vi "main.vi"() -> ()   [LabVIEW 2019]
uses:
  <vilib>/Utility/file.llb/Write Delimited Spreadsheet (string).vi
  <vilib>/Utility/file.llb/Read Delimited Spreadsheet (DBL).vi
panel:
  in  "设备名":tag="Dev11"
  out "行":i32
  out "列":i32
  in  "?":bool
  out "Log":string
  out "Load6":bool
  out "Load5":bool
  out "Load4":bool
  out "Load3":bool
  out "Load2":bool
  out "Load1":bool
  out "Load0":bool
  out "data":bool[](array[boolean]) caption="数据"
  # "测试报告状态："
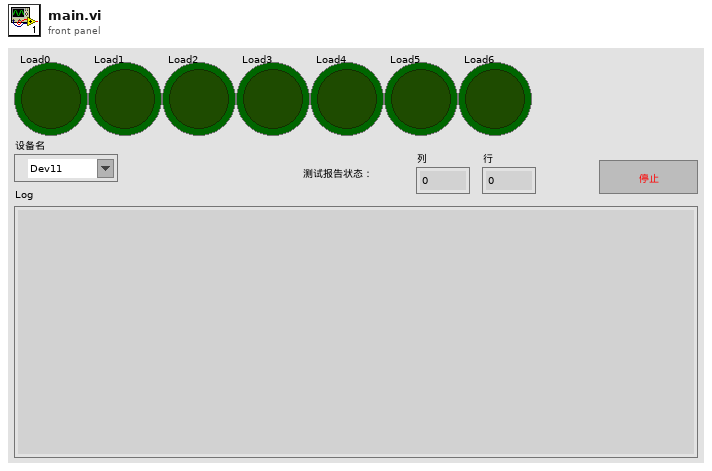
[diagram p1: front panel]
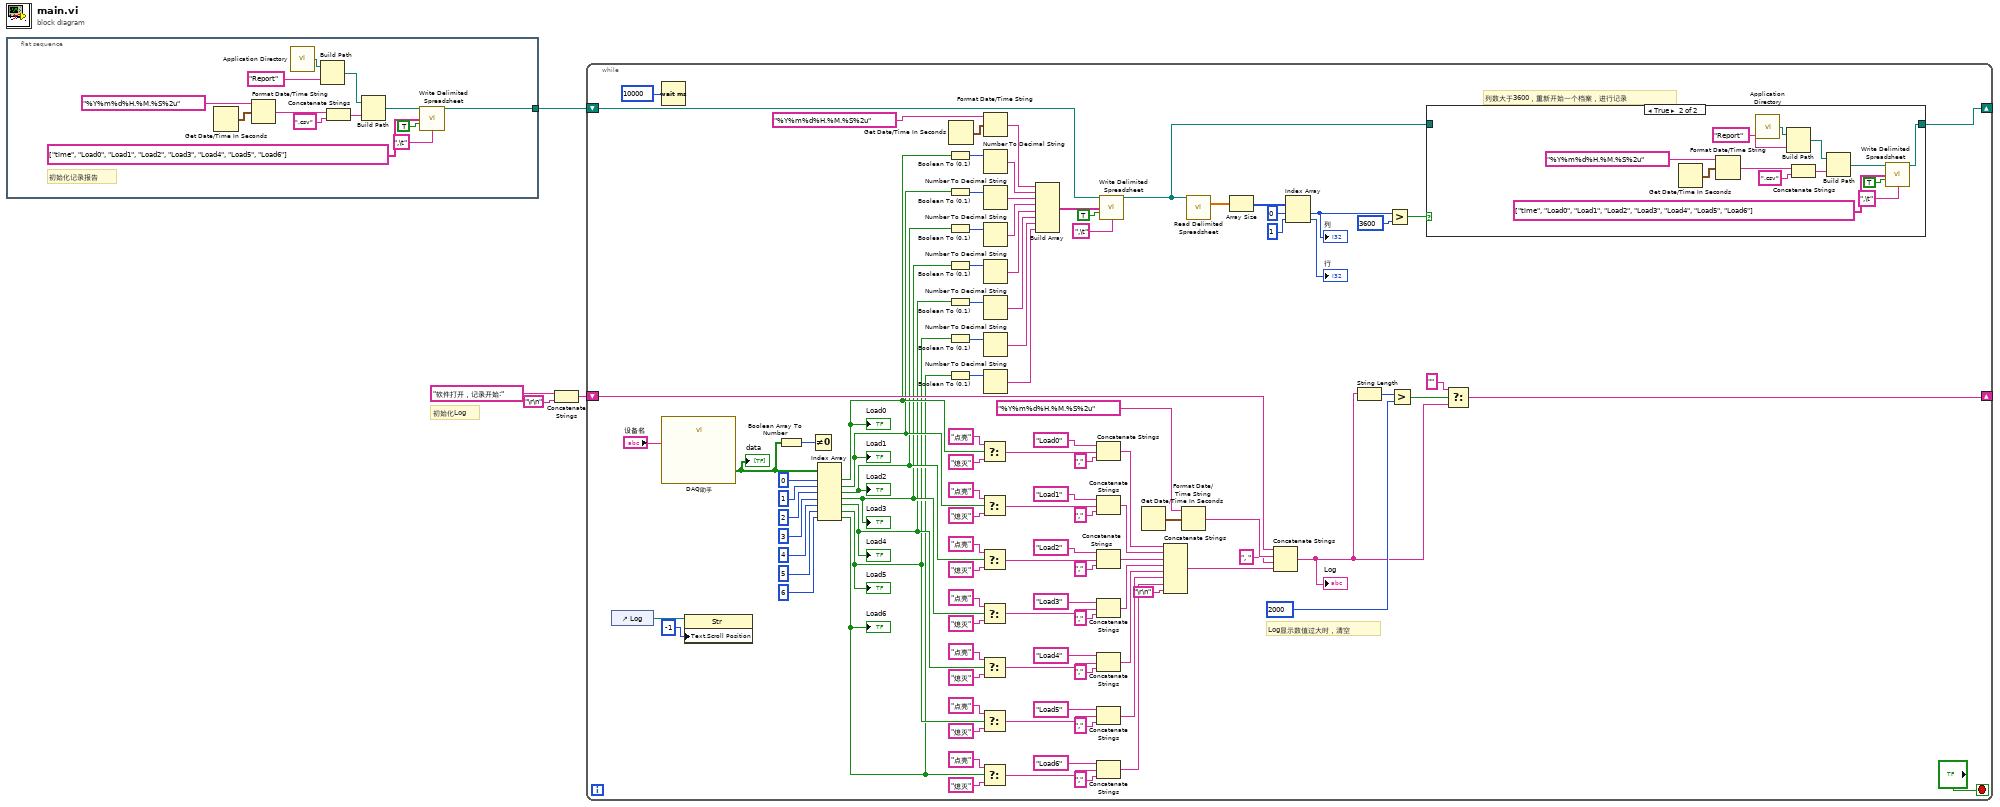
[diagram p0: block diagram]
diagram:
  # "初始化Log"
  n1 = flat-sequence {
    tunnel: [w5] -> w4
    frame #0 {
      # "初始化记录报告"
      n2 = Get Date/Time In Seconds() -> (seconds since 1Jan1904=w16:timestamp)
      n3 = Format Date/Time String(time format string (%c)="%Y%m%d%H.%M.%S%2u" ("时间格式字符串(%c)"), seconds (now)=w16) -> (date/time string=w17:string)  [unwired: 1 in]
      n4 = call <vilib>:"Application Directory.vi"() -> ("Application Directory"=w6:path)
      n5 = Build Path(base path=w6, name or relative path="Report" ("名称或相对路径")) -> (appended path=w9:path)
      n6 = Concatenate Strings(w17, ".csv" ("名称或相对路径")) -> (w13:string)
      n7 = Build Path(base path=w9, name or relative path=w13) -> (appended path=w10:path)
      n8 = call-poly <vilib>:"Write Delimited Spreadsheet.vi"("file path (dialog if empty)"=w10, "1D data"=string[] ["time", "Load0", "Load1", "Load2", "Load3", "Load4", "Load5", "Load6"], "append to file? (new file:F)"=TRUE, "delimiter (\\t)"=",\t" ("delimiter (\\t)")) -> ("new file path (Not A Path if cancelled)"=w5:path)  [unwired: 10 in, 1 out]
    }
  }
  n9 = Concatenate Strings("软件打开，记录开始:", "\r\n") -> (w1:string)
  n10 = while {
    shift-right: [w24] -> _
    shift-left: w1 -> [w73]
    shift-right: [w34] -> _
    shift-left: w4 -> [w69]
    stop <- "?" stop-if-true
    # "Log显示数值过大时，清空"
    # "列数大于3600，重新开始一个档案，进行记录"
    n11 = control-ref of="Log"() -> (w23:refnum<vi>)
    n12 = Wait (ms)(milliseconds to wait=u32 10000 ("等待时间（毫秒）")) -> ()  [unwired: 1 out]
    n13 = call "DAQ助手"("设备名"="设备名") -> ("data"=w117:bool[])  [unwired: 16 in, 2 out]
    "data" <- w117
    n14 = property class="Str"(reference=w23, "Text.Scroll Position"=-1 ("y")) -> ()  [unwired: 1 in, 2 out]
    n15 = Boolean Array To Number(Boolean array=w117) -> (number=w116:u32)
    n16 = Not Equal To 0?(x=w116) -> ()  [unwired: 1 out]
    n17 = Index Array(array=w117, index #1=0 ("索引"), index #2=1 ("索引"), index #3=2 ("索引"), index #4=3 ("索引"), index #5=4 ("索引"), index #6=5 ("索引"), index #7=6 ("索引")) -> (element #1=w68:bool, element #2=w60:bool, element #3=w59:bool, element #4=w58:bool, element #5=w57:bool, element #6=w56:bool, element #7=w55:bool)
    "Load0" <- w68
    "Load1" <- w60
    "Load2" <- w59
    "Load3" <- w58
    "Load4" <- w57
    "Load5" <- w56
    "Load6" <- w55
    n18 = Boolean To (0,1)(Boolean=w68) -> (0, 1=w67:i16)
    n19 = Boolean To (0,1)(Boolean=w60) -> (0, 1=w66:i16)
    n20 = Boolean To (0,1)(Boolean=w59) -> (0, 1=w64:i16)
    n21 = Boolean To (0,1)(Boolean=w58) -> (0, 1=w65:i16)
    n22 = Boolean To (0,1)(Boolean=w57) -> (0, 1=w61:i16)
    n23 = Boolean To (0,1)(Boolean=w56) -> (0, 1=w62:i16)
    n24 = Boolean To (0,1)(Boolean=w55) -> (0, 1=w63:i16)
    n25 = Get Date/Time In Seconds() -> (seconds since 1Jan1904=w53:timestamp)
    n26 = Select(t="点亮", s=w68, f="熄灭") -> (s? t:f=w112:string)
    n27 = Select(t="点亮", s=w60, f="熄灭") -> (s? t:f=w109:string)
    n28 = Select(t="点亮", s=w59, f="熄灭") -> (s? t:f=w99:string)
    n29 = Select(t="点亮", s=w58, f="熄灭") -> (s? t:f=w102:string)
    n30 = Select(t="点亮", s=w57, f="熄灭") -> (s? t:f=w84:string)
    n31 = Select(t="点亮", s=w56, f="熄灭") -> (s? t:f=w87:string)
    n32 = Select(t="点亮", s=w55, f="熄灭") -> (s? t:f=w92:string)
    n33 = Format Date/Time String(time format string (%c)="%Y%m%d%H.%M.%S%2u" ("时间格式字符串(%c)"), seconds (now)=w53) -> (date/time string=w52:string)  [unwired: 1 in]
    n34 = Number To Decimal String(number=w67) -> (decimal integer string=w51:string)  [unwired: 1 in]
    n35 = Number To Decimal String(number=w66) -> (decimal integer string=w50:string)  [unwired: 1 in]
    n36 = Number To Decimal String(number=w64) -> (decimal integer string=w49:string)  [unwired: 1 in]
    n37 = Number To Decimal String(number=w65) -> (decimal integer string=w48:string)  [unwired: 1 in]
    n38 = Number To Decimal String(number=w61) -> (decimal integer string=w47:string)  [unwired: 1 in]
    n39 = Number To Decimal String(number=w62) -> (decimal integer string=w46:string)  [unwired: 1 in]
    n40 = Number To Decimal String(number=w63) -> (decimal integer string=w45:string)  [unwired: 1 in]
    n41 = Build Array(w52, w51, w50, w49, w48, w47, w46, w45) -> (w43:string[])
    n42 = Concatenate Strings("Load0" ("字符串"), w112, "," ("字符串")) -> (w80:string)
    n43 = Concatenate Strings("Load1" ("字符串"), w109, "," ("字符串")) -> (w79:string)
    n44 = Concatenate Strings("Load2" ("字符串"), w99, "," ("字符串")) -> (w78:string)
    n45 = Concatenate Strings("Load3" ("字符串"), w102, "," ("字符串")) -> (w77:string)
    n46 = Concatenate Strings("Load4" ("字符串"), w84, "," ("字符串")) -> (w76:string)
    n47 = Concatenate Strings("Load5" ("字符串"), w87, "," ("字符串")) -> (w75:string)
    n48 = Concatenate Strings("Load6" ("字符串"), w92, "," ("字符串")) -> (w74:string)
    n49 = call-poly <vilib>:"Write Delimited Spreadsheet.vi"("file path (dialog if empty)"=w69, "1D data"=w43, "append to file? (new file:F)"=TRUE, "delimiter (\\t)"=",\t" ("delimiter (\\t)")) -> ("new file path (Not A Path if cancelled)"=w33:path)  [unwired: 10 in, 1 out]
    n50 = Get Date/Time In Seconds() -> (seconds since 1Jan1904=w32:timestamp)
    n51 = Concatenate Strings(w80, w79, w78, w77, w76, w75, w74, "\r\n") -> (w20:string)
    n52 = Format Date/Time String(time format string (%c)="%Y%m%d%H.%M.%S%2u" ("时间格式字符串(%c)"), seconds (now)=w32) -> (date/time string=w30:string)  [unwired: 1 in]
    n53 = call-poly <vilib>:"Read Delimited Spreadsheet.vi"("file path (dialog if empty)"=w33) -> ("all rows"=w41:dbl[][])  [unwired: 9 in, 5 out]
    n54 = Array Size(array=w41) -> (size(s)=w40:i32[])
    n55 = Concatenate Strings(w73, w30, ", " ("字符串"), w20) -> (w25:string)
    "Log" <- w25
    n56 = Index Array(array=w40, index #1=0 ("索引"), index #2=1 ("索引")) -> (element #1=w21:i32, element #2=→"行":i32)
    "列" <- w21
    n57 = String Length(string=w25) -> (length=w29:i32)
    n58 = Greater?(x=w21, y=3600) -> (0:w35:bool)
    n59 = Greater?(x=w29, y=2000) -> (0:w27:bool)
    n60 = case shown="True" w35 {
      tunnel: [w125 w126] -> w34
      tunnel: w33 -> [w125 _]
      frame False {
      }
      frame True {
        n61 = Get Date/Time In Seconds() -> (seconds since 1Jan1904=w128:timestamp)
        n62 = Format Date/Time String(time format string (%c)="%Y%m%d%H.%M.%S%2u" ("时间格式字符串(%c)"), seconds (now)=w128) -> (date/time string=w127:string)  [unwired: 1 in]
        n63 = call <vilib>:"Application Directory.vi"() -> ("Application Directory"=w138:path)
        n64 = Build Path(base path=w138, name or relative path="Report" ("名称或相对路径")) -> (appended path=w135:path)
        n65 = Concatenate Strings(w127, ".csv" ("名称或相对路径")) -> (w131:string)
        n66 = Build Path(base path=w135, name or relative path=w131) -> (appended path=w134:path)
        n67 = call-poly <vilib>:"Write Delimited Spreadsheet.vi"("file path (dialog if empty)"=w134, "1D data"=string[] ["time", "Load0", "Load1", "Load2", "Load3", "Load4", "Load5", "Load6"], "append to file? (new file:F)"=TRUE, "delimiter (\\t)"=",\t" ("delimiter (\\t)")) -> ("new file path (Not A Path if cancelled)"=w126:path)  [unwired: 10 in, 1 out]
      }
    }
    n68 = Select(t="" ("时间格式字符串(%c)"), s=w27, f=w25) -> (s? t:f=w24:string)
  }
